vi "DI Read_TS_v2.vi"(8 "error in (no error)":errorcluster, 11 "ControlBoard VISA":refnum<visa-resource-name>="ControlBoard") -> (0 "error out":errorcluster, 1 "DI Reading (Hex String)":string, 2 "DI Reading":bool[](array[boolean]), 3 "VISA Refnum out":refnum<visa-resource-name>)   [LabVIEW 2022 SP3]
uses:
  SupportVIs/VISA Flush IO Buffer Mask.ctl
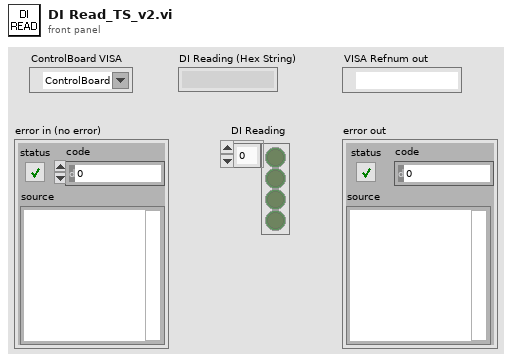
[diagram p1: front panel]
types:
  T1 = typedef "VISA Flush IO Buffer Mask.ctl" = u16
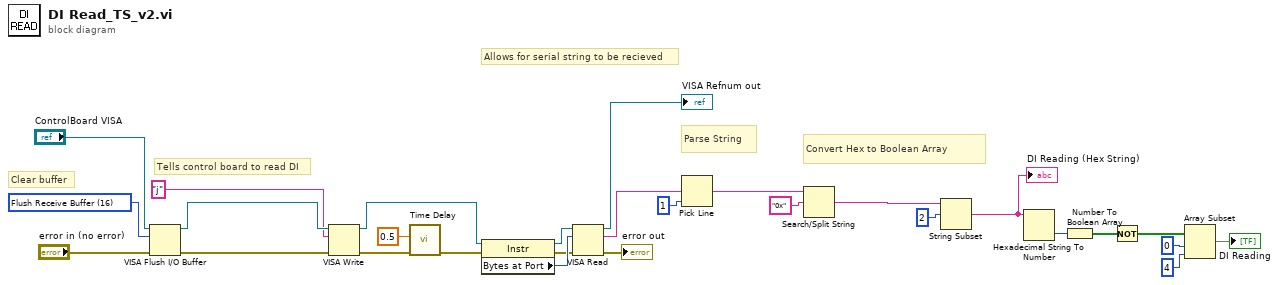
[diagram p0: block diagram]
diagram:
  w18 = T1 16 items=["Flush Receive Buffer"=16, "Write Transmit Buffer to Device"=32, "Flush Receive Buffer (No I/O)"=64, "Flush Transmit Buffer"=128] ("Mask")
  # "Convert Hex to Boolean Array"
  # "Clear buffer"
  # "Parse String"
  # "Allows for serial string to be recieved"
  # "Tells control board to read DI"
  n1 = VISA Flush I/O Buffer(VISA resource name="ControlBoard VISA", mask (16)=w18, error in (no error)="error in (no error)") -> (VISA resource name out=w20:refnum<visa-resource-name>, error out=w1:errorcluster)
  n2 = VISA Write(VISA resource name=w20, write buffer="j", error in (no error)=w1) -> (VISA resource name out=w22:refnum<visa-resource-name>, error out=w19:errorcluster)  [unwired: 1 out]
  n3 = call "Time Delay"("error in (no error)"=w19, "Delay Time (s)"=0.5) -> ("error out"=w21:errorcluster)  [unwired: 9 in]
  n4 = property class="Instr"(reference=w22, error in=w21) -> (reference out=w15:refnum<visa-resource-name>, error out=w16:errorcluster, "Bytes at Port"=w17:u32)
  n5 = VISA Read(VISA resource name=w15, byte count=w17, error in (no error)=w16) -> (VISA resource name out=→"VISA Refnum out":refnum<visa-resource-name>, read buffer=w26:string, error out=→"error out":errorcluster)  [unwired: 1 out]
  n6 = Pick Line(multi-line string=w26, line index=1) -> (output string=w27:string)  [unwired: 1 in]
  n7 = Search/Split String(string=w27, search string/char (-)="0x" ("regular expression")) -> (match + rest of string=w24:string)  [unwired: 1 in, 2 out]
  n8 = String Subset(string=w24, offset (0)=2) -> (substring=w9:string)  [unwired: 1 in]
  "DI Reading (Hex String)" <- w9
  n9 = Hexadecimal String To Number(string=w9) -> (number=w11:u32)  [unwired: 2 in, 1 out]
  n10 = Number To Boolean Array(number=w11) -> (Boolean array=w10:bool[])
  n11 = Not(x=w10) -> (.not. x?=w6:bool[])
  n12 = Array Subset(array=w6, index=0, length=4) -> (→"DI Reading":bool[])
